vi "FTW-Example-EventLogger.vi"() -> ()   [LabVIEW 2014]
uses:
  src/core/actor/logger/FTW-Logger.lvclass
panel:
  in  "Logger Configuration":string="{\n  \"Identity\": \"EventLog\",\n  \"InboxAddress\": \"tcp://127.0.0.1:*\",\n  \"PublisherAddress\": \"\",\n  \"DebugShowPanel\": false,\n  \"DebugEnableInboxLogging\": false,\n  \"DebugEnableJobLogging\": false,\n  \"ApplicationName\": \"LoggerExample\",\n  \"LoggerDirectory\": \"[UserDesktop]\\\\Logs\",\n  \"LoggerDiskThrashDelay\": 200\n}"
  out "error out":errorcluster
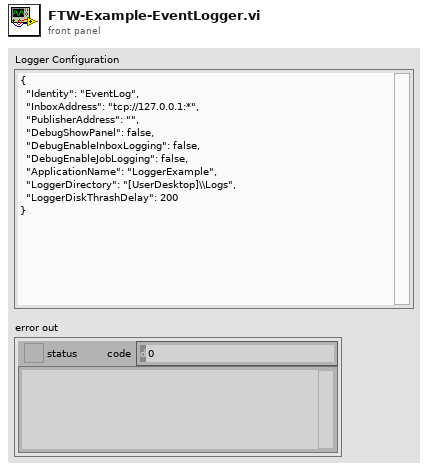
[diagram p1: front panel]
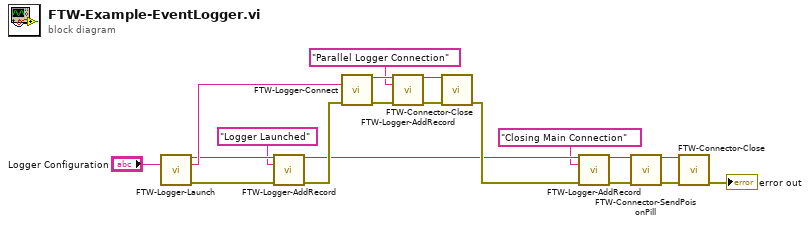
[diagram p0: block diagram]
diagram:
  n1 = call "FTW-Logger-Launch.vi"("FTW Logger Configuration"="Logger Configuration") -> ("FTW Logger Connector"=w13:refnum<class "FTW-Logger.lvclass">, "Logger Address"=w15:string, "error out"=w12:errorcluster)  [unwired: 12 in]
  n2 = call "FTW-Logger-AddRecord.vi"("FTW Logger Connector"=w13, "Event Type"="Logger Launched", "error in"=w12) -> ("FTW Logger Connector out"=w7:refnum<class "FTW-Logger.lvclass">, "error out"=w11:errorcluster)  [unwired: 10 in, 1 out]
  n3 = call "FTW-Logger-Connect.vi"("Logger Address"=w15, "error in"=w11) -> ("FTW Logger Connector"=w18:refnum<class "FTW-Logger.lvclass">, "error out"=w16:errorcluster)  [unwired: 12 in]
  n4 = call "FTW-Logger-AddRecord.vi"("FTW Logger Connector"=w18, "Event Type"="Parallel Logger Connection", "error in"=w16) -> ("FTW Logger Connector out"=w9:refnum<class "FTW-Logger.lvclass">, "error out"=w8:errorcluster)  [unwired: 10 in, 1 out]
  n5 = call-dynamic "FTW-Connector-Close.vi"("FTW Actor Connector"=w9, "error in"=w8) -> ("error out"=w19:errorcluster)  [unwired: 13 in]
  n6 = call "FTW-Logger-AddRecord.vi"("FTW Logger Connector"=w7, "Event Type"="Closing Main Connection", "error in"=w19) -> ("FTW Logger Connector out"=w5:refnum<class "FTW-Logger.lvclass">, "error out"=w4:errorcluster)  [unwired: 10 in, 1 out]
  n7 = call-dynamic "FTW-Connector-SendPoisonPill.vi"("FTW Actor Connector"=w5, "error in"=w4) -> ("FTW Actor Connector out"=w3:refnum<class "FTW-Logger.lvclass">, "error out"=w2:errorcluster)  [unwired: 10 in, 2 out]
  n8 = call-dynamic "FTW-Connector-Close.vi"("FTW Actor Connector"=w3, "error in"=w2) -> ("error out"=→"error out":errorcluster)  [unwired: 13 in]
